vi "TestBench.vi"() -> ()   [LabVIEW 2015, in "TestBench.lvlib"]
uses:
  TestBench.lvlib
  TestBenchData.ctl
  TestBenchState.ctl
  <vilib>/DAQmx/read.llb/DAQmx Read (Analog DBL 1Chan 1Samp).vi
  <vilib>/DAQmx/write.llb/DAQmx Write (Analog 2D DBL NChan NSamp).vi
  <vilib>/DAQmx/read.llb/DAQmx Read (Analog 1D DBL 1Chan NSamp).vi
  <vilib>/DAQmx/write.llb/DAQmx Write (Digital 1D Bool NChan 1Samp 1Line).vi
  <vilib>/DAQmx/create/channels.llb/DAQmx Create Channel (AI-Current-Basic).vi
  <vilib>/DAQmx/miscellaneous.llb/DAQmx Fill In Error Info.vi
  TestBenchVariables.vi
  <vilib>/DAQmx/create/channels.llb/DAQmx Create Channel (AO-Voltage-Basic).vi
  <vilib>/DAQmx/configure/timing.llb/DAQmx Timing (Sample Clock).vi
  <vilib>/DAQmx/create/channels.llb/DAQmx Create Channel (AI-Voltage-Basic).vi
  <vilib>/DAQmx/create/channels.llb/DAQmx Create Channel (DO-Digital Output).vi
  <resource>/objmgr/daqmx.rc
  <vilib>/Analysis/NI_AALPro.lvlib
panel:
  out "Quit DMM":bool
  in  "index (row)":i32=1
  out "Waveform Graph":dbl[](graph)
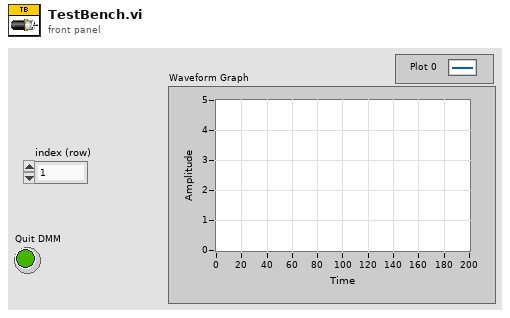
[diagram p1: front panel]
types:
  T1 = typedef "TestBench.lvlib/TestBenchState.ctl" = enum16{"Init", "Loop", "Check Errors", "Reset", "Close"}
  T2 = typedef "TestBench.lvlib/TestBenchData.ctl" = cluster{"AO PWMs":refnum<k21>, "AI Enkoder":refnum<k21>, "DOs":refnum<k21>, "AI Buffer":dbl[]}
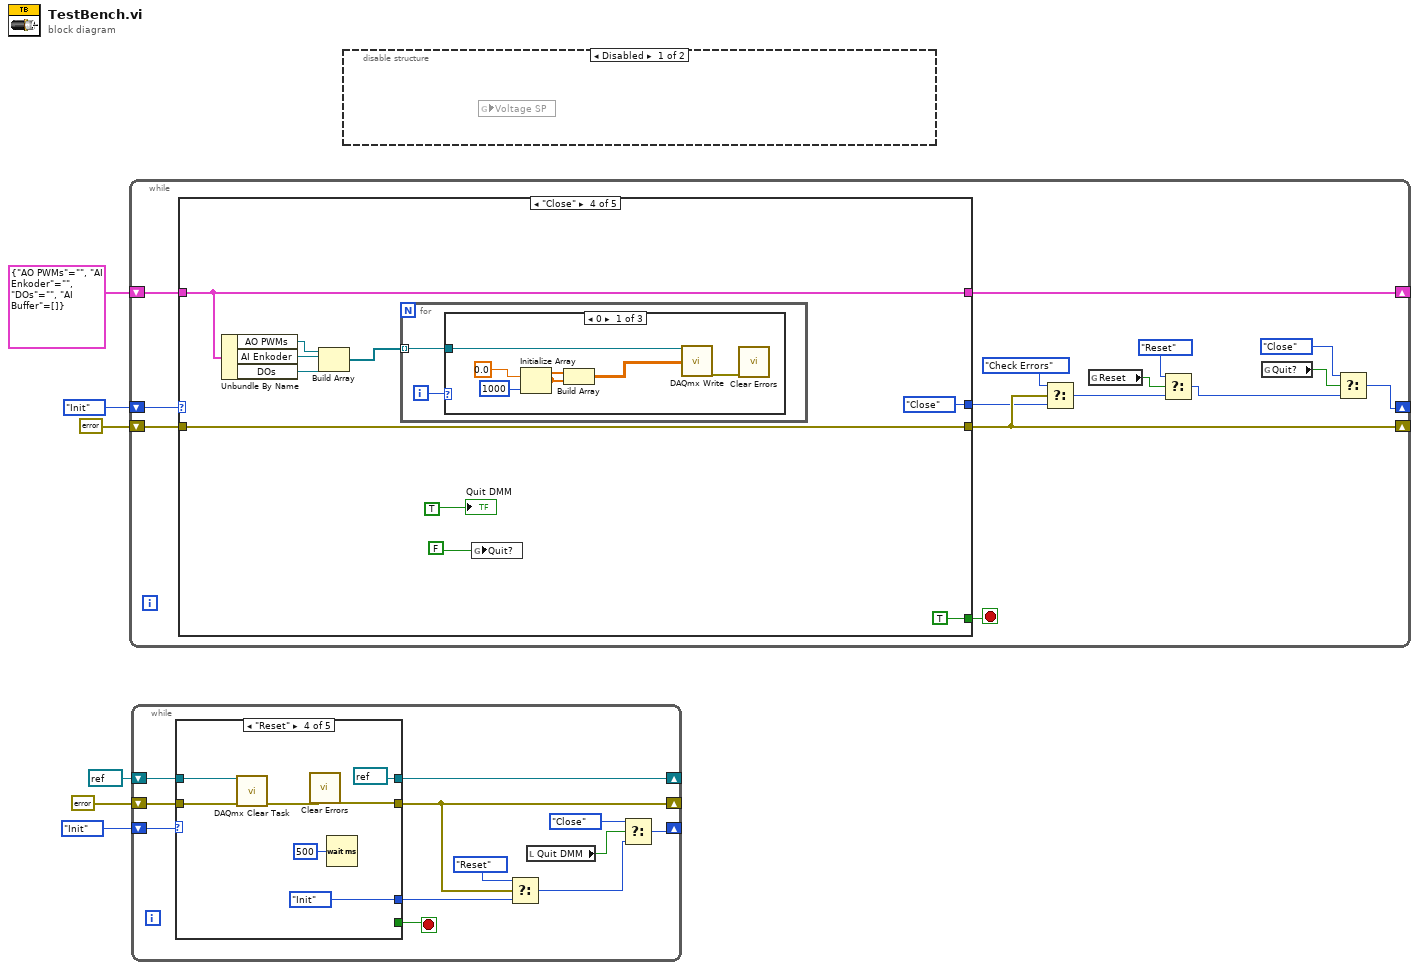
[diagram p0: block diagram]
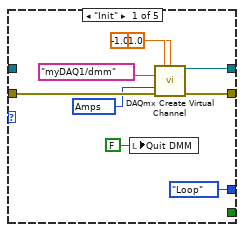
[diagram p2: hidden frame]
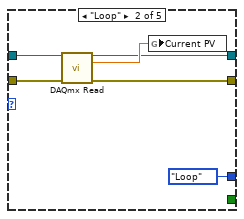
[diagram p3: hidden frame]
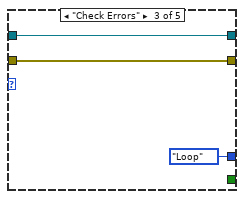
[diagram p4: hidden frame]
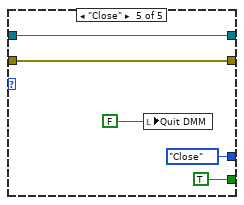
[diagram p5: hidden frame]
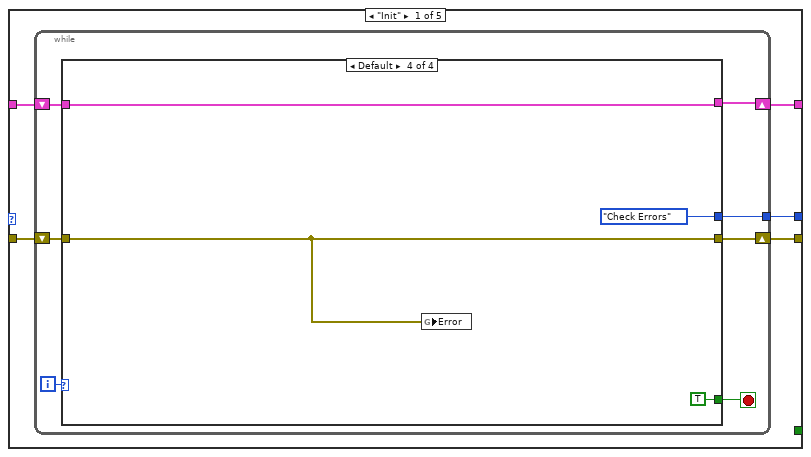
[diagram p7: hidden frame]
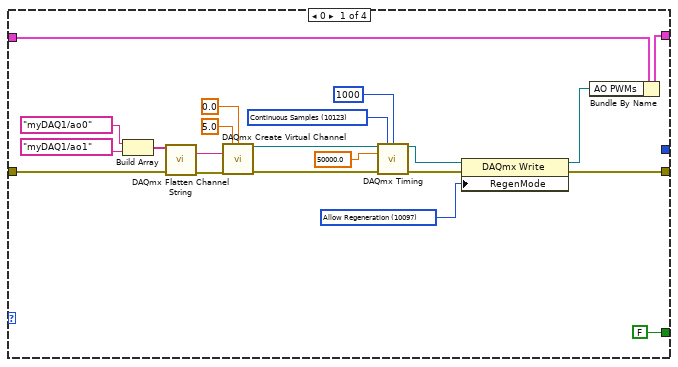
[diagram p8: hidden frame]
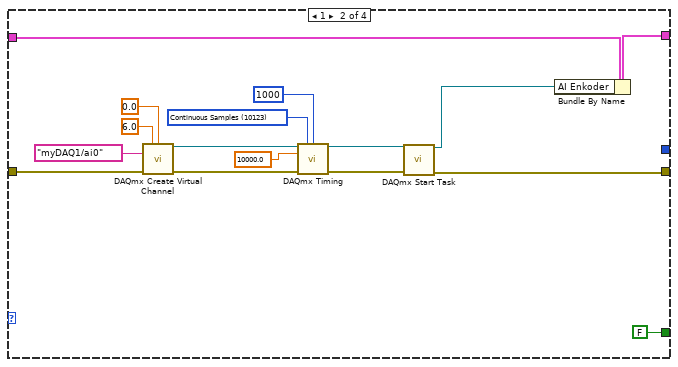
[diagram p9: hidden frame]
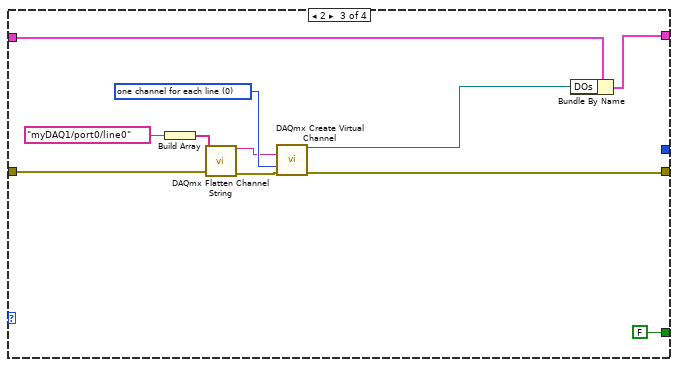
[diagram p10: hidden frame]
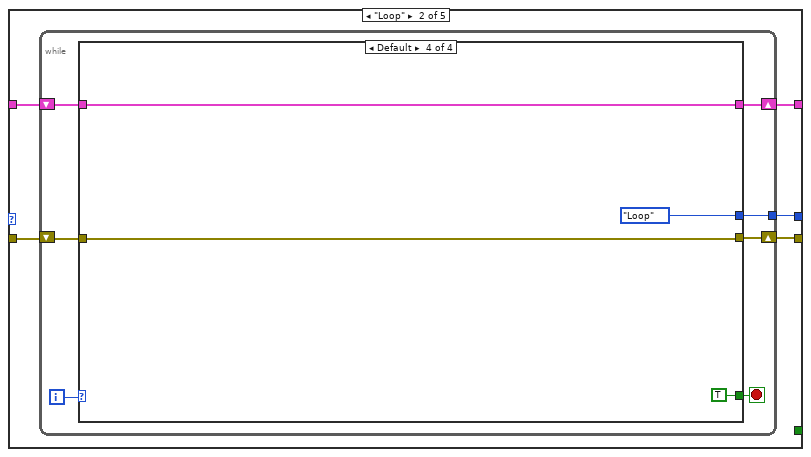
[diagram p11: hidden frame]
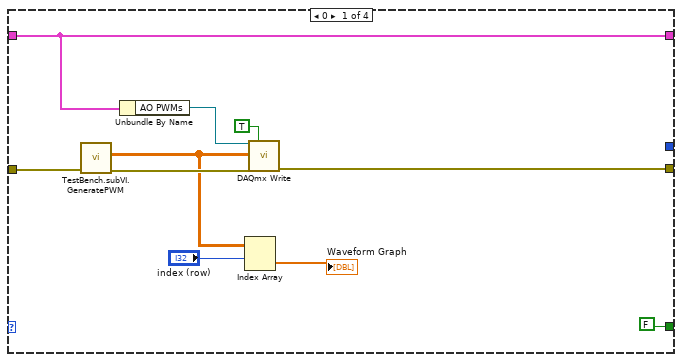
[diagram p12: hidden frame]
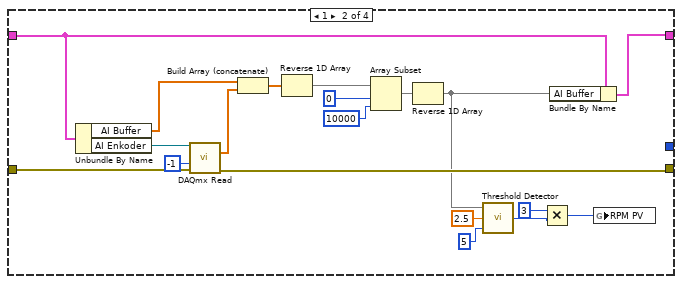
[diagram p13: hidden frame]
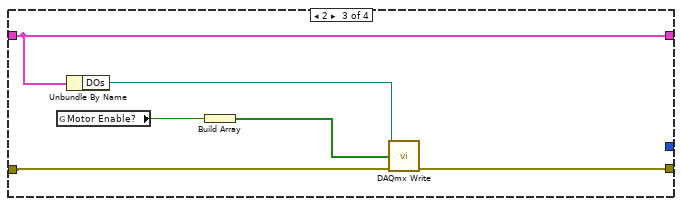
[diagram p14: hidden frame]
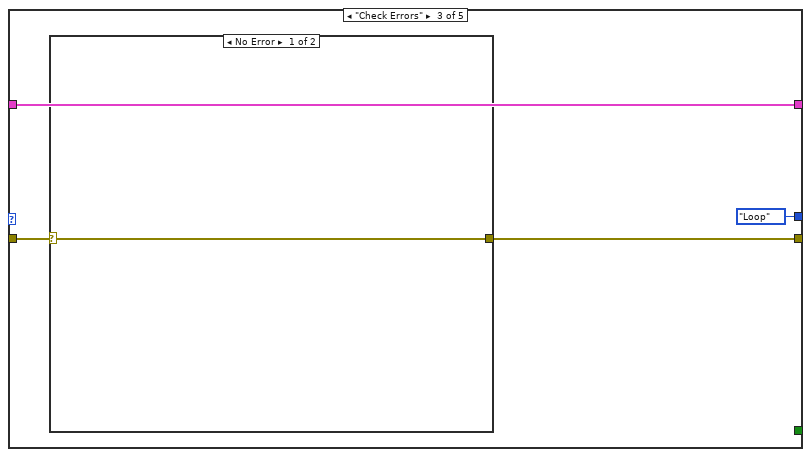
[diagram p15: hidden frame]
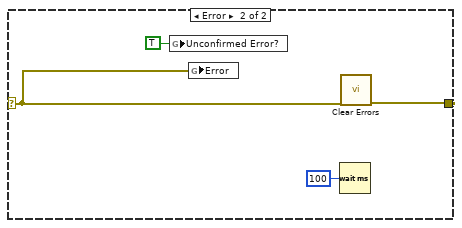
[diagram p16: hidden frame]
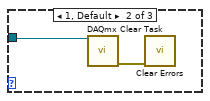
[diagram p17: hidden frame]
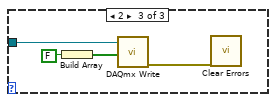
[diagram p18: hidden frame]
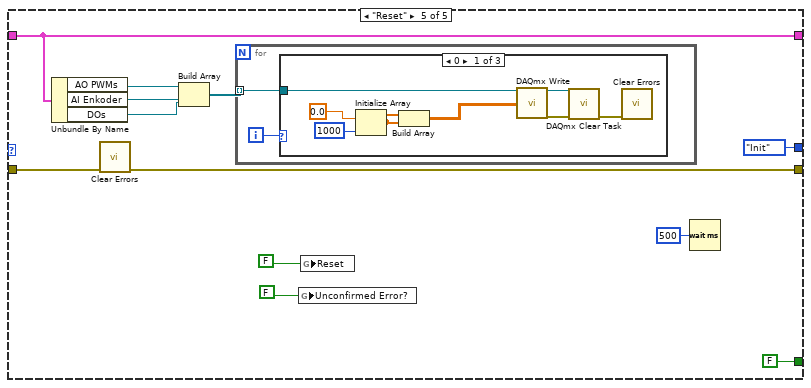
[diagram p19: hidden frame]
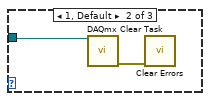
[diagram p20: hidden frame]
diagram:
  n1 = while {
    shift-right: [w7] -> _
    shift-left: TestBenchState."Init" -> [w21]
    shift-right: [w19] -> _
    shift-left: T2 {"AO PWMs"="", "AI Enkoder"="", "DOs"="", "AI Buffer"=[]} -> [w20]
    shift-right: [w15] -> _
    shift-left: errorcluster {"status"=FALSE, "code"=0, "source"=""} ("error out") -> [w18]
    stop <- w12 stop-if-true
    n2 = case shown="\"Close\"" w21 {
      tunnel: w20 -> [w26 w90 w138 w153 w172]
      tunnel: [w25 w86 w138 w153 w172] -> w19
      tunnel: [w24 w87 TestBenchState."Loop" TestBenchState."Close" TestBenchState."Init"] -> w14
      tunnel: [w23 w88 w139 w154 w170] -> w15
      tunnel: w18 -> [w22 w89 w140 w154 w171]
      tunnel: [_ _ _ TRUE FALSE] -> w12
      frame "Init" {
        n3 = while {
          shift-right: [w31] -> w25
          shift-left: w26 -> [w32]
          shift-right: [w28] -> w23
          shift-left: w22 -> [w29]
          tunnel: [w27] -> w24
          i -> [w33]
          stop <- w30 stop-if-true
          n4 = case shown="Default" w33 {
            tunnel: w32 -> [w48 w68 w81 w84]
            tunnel: [w47 w67 w80 w84] -> w31
            tunnel: [FALSE FALSE FALSE TRUE] -> w30
            tunnel: w29 -> [w39 w59 w75 w82]
            tunnel: [w35 w56 w76 w82] -> w28
            tunnel: [_ _ _ TestBenchState."Check Errors"] -> w27
            frame 0 {
              w37 = 10097 items=["Allow Regeneration"=10097, "Do Not Allow Regeneration"=10158] ("RegenMode")
              w43 = 10123 items=["Finite Samples"=10178, "Continuous Samples"=10123, "Hardware Timed Single Point"=12522] ("sample mode")
              n5 = Build Array(tag "myDAQ1/ao0" ("physical channels"), tag "myDAQ1/ao1" ("physical channels")) -> (w50:tag[])
              n6 = call <vilib>:"DAQmx Flatten Channel String.vi"("names in"=w50, "error in"=w39) -> ("names out"=w49:string, "error out"=w45:errorcluster)  [unwired: 12 in]
              n7 = call-poly <vilib>:"DAQmx Create Virtual Channel.vi"("maximum value"=5.0, "minimum value"=0.0, "physical channels"=w49, "error in"=w45) -> ("task out"=w41:refnum<k21>, "error out"=w44:errorcluster)  [unwired: 10 in]
              n8 = call-poly <vilib>:"DAQmx Timing.vi"("task/channels in"=w41, "sample mode"=w43, "samples per channel"=1000, "rate"=50000.0, "error in"=w44) -> ("task out"=w38:refnum<k21>, "error out"=w36:errorcluster)  [unwired: 9 in]
              n9 = property class="DAQmx Write"(reference=w38, error in=w36, "RegenMode"=w37) -> (reference out=w34:refnum<k21>, error out=w35:errorcluster)
              n10 = Bundle By Name(cluster=w48, "AO PWMs"=w34) -> (w47:T2)
            }
            frame 1 {
              w64 = 10123 items=["Finite Samples"=10178, "Continuous Samples"=10123, "Hardware Timed Single Point"=12522] ("sample mode")
              n11 = call-poly <vilib>:"DAQmx Create Virtual Channel.vi"("maximum value"=6.0, "minimum value"=0.0, "physical channels"=tag "myDAQ1/ai0", "error in"=w59) -> ("task out"=w62:refnum<k21>, "error out"=w65:errorcluster)  [unwired: 10 in]
              n12 = call-poly <vilib>:"DAQmx Timing.vi"("task/channels in"=w62, "sample mode"=w64, "samples per channel"=1000, "rate"=10000.0, "error in"=w65) -> ("task out"=w57:refnum<k21>, "error out"=w58:errorcluster)  [unwired: 9 in]
              n13 = call <vilib>:"DAQmx Start Task.vi"("task/channels in"=w57, "error in"=w58) -> ("task out"=w55:refnum<k21>, "error out"=w56:errorcluster)  [unwired: 12 in]
              n14 = Bundle By Name(cluster=w68, "AI Enkoder"=w55) -> (w67:T2)
            }
            frame 2 {
              w78 = 0 items=["one channel for each line", "one channel for all lines"] ("line grouping")
              n15 = Build Array(tag "myDAQ1/port0/line0" ("lines")) -> (w73:tag[])
              n16 = call <vilib>:"DAQmx Flatten Channel String.vi"("names in"=w73, "error in"=w75) -> ("names out"=w72:string, "error out"=w71:errorcluster)  [unwired: 12 in]
              n17 = call-poly <vilib>:"DAQmx Create Virtual Channel.vi"("lines"=w72, "line grouping"=w78, "error in"=w71) -> ("task out"=w77:refnum<k21>, "error out"=w76:errorcluster)  [unwired: 11 in]
              n18 = Bundle By Name(cluster=w81, "DOs"=w77) -> (w80:T2)
            }
            frame Default {
              n19 = global write "TestBenchVariables.vi" "Error"(w82) -> ()
            }
          }
        }
      }
      frame "Loop" {
        n20 = while {
          shift-right: [w91] -> w86
          shift-left: w90 -> [w95]
          tunnel: [w92] -> w87
          shift-right: [w93] -> w88
          shift-left: w89 -> [w94]
          i -> [w97]
          stop <- w96 stop-if-true
          n21 = case shown="Default" w97 {
            tunnel: [FALSE _ _ TRUE] -> w96
            tunnel: w95 -> [w102 w116 w127 w136]
            tunnel: w94 -> [w106 w122 w129 w135]
            tunnel: [w103 w114 w128 w135] -> w93
            tunnel: [w102 w115 w127 w136] -> w91
            tunnel: [_ _ _ TestBenchState."Loop"] -> w92
            frame 0 {
              n22 = call "TestBench.subVI.GeneratePWM.vi"("error in (no error)"=w106) -> ("error out"=w105:errorcluster, "PWMs"=w101:dbl[][])  [unwired: 9 in]
              n23 = Unbundle By Name(w102) -> ("AO PWMs"=w98:refnum<k21>)
              n24 = Index Array(array=w101, index (row)="index (row)") -> (element=→"Waveform Graph":dbl[])  [unwired: 1 in]
              n25 = call-poly <vilib>:"DAQmx Write.vi"("task/channels in"=w98, "auto start"=TRUE, "data"=w101, "error in"=w105) -> ("error out"=w103:errorcluster)  [unwired: 9 in, 2 out]
            }
            frame 1 {
              n26 = Unbundle By Name(w116) -> ("AI Buffer"=w119:dbl[], "AI Enkoder"=w121:refnum<k21>)
              n27 = call-poly <vilib>:"DAQmx Read.vi"("task/channels in"=w121, "number of samples per channel"=-1, "error in"=w122) -> ("data"=w118:dbl[], "error out"=w114:errorcluster)  [unwired: 10 in, 1 out]
              n28 = Build Array (concatenate)(w119, w118) -> (w126:dbl[])
              n29 = Reverse 1D Array(array=w126) -> (reversed array=w117:dbl[])
              n30 = Array Subset(array=w117, index=0, length=10000) -> (w125:dbl[])
              n31 = Reverse 1D Array(array=w125) -> (reversed array=w111:dbl[])
              n32 = call <vilib>:"Threshold Detector.vi"("width"=5, "threshold"=2.5, "X"=w111) -> ("count"=w110:i32)  [unwired: 2 out]
              n33 = Multiply(x=3, y=w110) -> (x*y=w108:i32)
              n34 = Bundle By Name(cluster=w116, "AI Buffer"=w111) -> (w115:T2)
              n35 = global write "TestBenchVariables.vi" "RPM PV"(w108) -> ()
            }
            frame 2 {
              n36 = global read "TestBenchVariables.vi" "Motor Enable?"() -> (w132:bool)
              n37 = Unbundle By Name(w127) -> ("DOs"=w130:refnum<k21>)
              n38 = Build Array(w132) -> (w131:bool[])
              n39 = call-poly <vilib>:"DAQmx Write.vi"("task/channels in"=w130, "data"=w131, "error in"=w129) -> ("error out"=w128:errorcluster)  [unwired: 10 in, 2 out]
            }
            frame Default {
            }
          }
        }
      }
      frame "Check Errors" {
        n40 = case shown="No Error" w140 {
          selector: w140 -> [w141 w144]
          tunnel: [w141 w143] -> w139
          frame No Error {
          }
          frame Error {
            n41 = global write "TestBenchVariables.vi" "Unconfirmed Error?"(TRUE ("Unconfirmed Error?")) -> ()
            n42 = global write "TestBenchVariables.vi" "Error"(w144) -> ()
            n43 = Wait (ms)(milliseconds to wait=u32 100) -> ()  [unwired: 1 out]
            n44 = call <vilib>:"Clear Errors.vi"("error in (no error)"=w144) -> ("error out"=w143:errorcluster)  [unwired: 5 in, 1 out]
          }
        }
      }
      frame "Close" {
        n45 = Unbundle By Name(w153) -> ("AO PWMs"=w150:refnum<k21>, "AI Enkoder"=w149:refnum<k21>, "DOs"=w148:refnum<k21>)
        n46 = Build Array(w150, w149, w148) -> (w147:refnum<k21>[])
        n47 = for {
          tunnel: w147 -> [w156] mode=indexing
          i -> [w157]
          n48 = case shown="0" w157 {
            tunnel: w156 -> [w160 w164 w169]
            frame 0 {
              n49 = Initialize Array(0.0 ("element"), 1000 ("dimension size")) -> (w163:dbl[])
              n50 = Build Array(w163, w163) -> (w159:dbl[][])
              n51 = call-poly <vilib>:"DAQmx Write.vi"("task/channels in"=w160, "data"=w159) -> ("error out"=w158:errorcluster)  [unwired: 11 in, 2 out]
              n52 = call <vilib>:"Clear Errors.vi"("error in (no error)"=w158) -> ()  [unwired: 5 in, 2 out]
            }
            frame 1, Default {
              n53 = call <vilib>:"DAQmx Clear Task.vi"("task in"=w164) -> ("error out"=w165:errorcluster)  [unwired: 14 in]
              n54 = call <vilib>:"Clear Errors.vi"("error in (no error)"=w165) -> ()  [unwired: 5 in, 2 out]
            }
            frame 2 {
              n55 = Build Array(FALSE) -> (w167:bool[])
              n56 = call-poly <vilib>:"DAQmx Write.vi"("task/channels in"=w169, "data"=w167) -> ("error out"=w166:errorcluster)  [unwired: 11 in, 2 out]
              n57 = call <vilib>:"Clear Errors.vi"("error in (no error)"=w166) -> ()  [unwired: 5 in, 2 out]
            }
          }
        }
        n58 = global write "TestBenchVariables.vi" "Quit?"(FALSE) -> ()
        "Quit DMM" <- TRUE
      }
      frame "Reset" {
        n59 = Unbundle By Name(w172) -> ("AO PWMs"=w180:refnum<k21>, "AI Enkoder"=w179:refnum<k21>, "DOs"=w178:refnum<k21>)
        n60 = call <vilib>:"Clear Errors.vi"("error in (no error)"=w171) -> ("error out"=w170:errorcluster)  [unwired: 5 in, 1 out]
        n61 = Build Array(w180, w179, w178) -> (w175:refnum<k21>[])
        n62 = for {
          tunnel: w175 -> [w182] mode=indexing
          i -> [w183]
          n63 = case shown="0" w183 {
            tunnel: w182 -> [w188 w192 w199]
            frame 0 {
              n64 = Initialize Array(0.0 ("element"), 1000 ("dimension size")) -> (w191:dbl[])
              n65 = Build Array(w191, w191) -> (w187:dbl[][])
              n66 = call-poly <vilib>:"DAQmx Write.vi"("task/channels in"=w188, "data"=w187) -> ("task out"=w184:refnum<k21>, "error out"=w186:errorcluster)  [unwired: 11 in, 1 out]
              n67 = call <vilib>:"DAQmx Clear Task.vi"("task in"=w184, "error in"=w186) -> ("error out"=w185:errorcluster)  [unwired: 13 in]
              n68 = call <vilib>:"Clear Errors.vi"("error in (no error)"=w185) -> ()  [unwired: 5 in, 2 out]
            }
            frame 1, Default {
              n69 = call <vilib>:"DAQmx Clear Task.vi"("task in"=w192) -> ("error out"=w193:errorcluster)  [unwired: 14 in]
              n70 = call <vilib>:"Clear Errors.vi"("error in (no error)"=w193) -> ()  [unwired: 5 in, 2 out]
            }
            frame 2 {
              n71 = Build Array(FALSE) -> (w197:bool[])
              n72 = call-poly <vilib>:"DAQmx Write.vi"("task/channels in"=w199, "data"=w197) -> ("task out"=w196:refnum<k21>, "error out"=w195:errorcluster)  [unwired: 11 in, 1 out]
              n73 = call <vilib>:"DAQmx Clear Task.vi"("task in"=w196, "error in"=w195) -> ("error out"=w194:errorcluster)  [unwired: 13 in]
              n74 = call <vilib>:"Clear Errors.vi"("error in (no error)"=w194) -> ()  [unwired: 5 in, 2 out]
            }
          }
        }
        n75 = global write "TestBenchVariables.vi" "Unconfirmed Error?"(FALSE) -> ()
        n76 = global write "TestBenchVariables.vi" "Reset"(FALSE) -> ()
        n77 = Wait (ms)(milliseconds to wait=u32 500) -> ()  [unwired: 1 out]
      }
    }
    n78 = Select(t=TestBenchState."Check Errors", s=w15, f=w14) -> (s? t:f=w11:T1)
    n79 = global read "TestBenchVariables.vi" "Reset"() -> (w10:bool)
    n80 = Select(t=TestBenchState."Reset", s=w10, f=w11) -> (s? t:f=w8:T1)
    n81 = global read "TestBenchVariables.vi" "Quit?"() -> (w17:bool)
    n82 = Select(t=TestBenchState."Close", s=w17, f=w8) -> (s? t:f=w7:T1)
  }
  n83 = while {
    shift-right: [w211] -> _
    shift-left: refnum<k21> refnum ("task out") -> [w209]
    shift-right: [w207] -> _
    shift-left: errorcluster {"status"=FALSE, "code"=0, "source"=""} ("error out") -> [w202]
    shift-right: [w203] -> _
    shift-left: TestBenchState."Init" -> [w210]
    stop <- w201 stop-if-true
    n84 = case shown="\"Reset\"" w210 {
      tunnel: [w219 w224 w229 refnum<k21> refnum ("task out") w240] -> w211
      tunnel: w209 -> [_ w226 w229 w236 w240]
      tunnel: [w217 w223 w228 w232 w239] -> w207
      tunnel: [TestBenchState."Loop" TestBenchState."Loop" TestBenchState."Loop" TestBenchState."Init" TestBenchState."Close"] -> w206
      tunnel: w202 -> [w218 w221 w228 w235 w239]
      tunnel: [_ _ _ _ TRUE] -> w201
      frame "Init" {
        w214 = 10342 items=["Amps"=10342, "From Custom Scale"=10065] ("units")
        n85 = local write "Quit DMM"(FALSE ("Quit DMM")) -> ()
        n86 = call-poly <vilib>:"DAQmx Create Virtual Channel.vi"("maximum value"=1.0, "minimum value"=-1.0, "physical channels"=tag "myDAQ1/dmm", "units"=w214, "error in"=w218) -> ("task out"=w219:refnum<k21>, "error out"=w217:errorcluster)  [unwired: 9 in]
      }
      frame "Loop" {
        n87 = call-poly <vilib>:"DAQmx Read.vi"("task/channels in"=w226, "error in"=w221) -> ("task out"=w224:refnum<k21>, "data"=w225:dbl, "error out"=w223:errorcluster)  [unwired: 11 in]
        n88 = global write "TestBenchVariables.vi" "Current PV"(w225) -> ()
      }
      frame "Check Errors" {
      }
      frame "Reset" {
        n89 = call <vilib>:"DAQmx Clear Task.vi"("task in"=w236, "error in"=w235) -> ("error out"=w234:errorcluster)  [unwired: 13 in]
        n90 = call <vilib>:"Clear Errors.vi"("error in (no error)"=w234) -> ("error out"=w232:errorcluster)  [unwired: 5 in, 1 out]
        n91 = Wait (ms)(milliseconds to wait=u32 500) -> ()  [unwired: 1 out]
      }
      frame "Close" {
        n92 = local write "Quit DMM"(FALSE) -> ()
      }
    }
    n93 = Select(t=TestBenchState."Reset", s=w207, f=w206) -> (s? t:f=w204:T1)
    n94 = local read "Quit DMM"() -> (w200:bool)
    n95 = Select(t=TestBenchState."Close", s=w200, f=w204) -> (s? t:f=w203:T1)
  }
  n96 = disable-structure shown="Disabled" {
    frame Disabled {
      n97 = global read "TestBenchVariables.vi" "Voltage SP"() -> ()  [unwired: 1 in]
    }
    frame Enabled {
    }
  }
